vi "vipbBuild.vi"() -> (0 "error out":errorcluster)   [LabVIEW 2014, in "vipm-build-tools.lvlib"]
uses:
  vipm-build-tools.lvlib
  <vilib>/Utility/error.llb/DialogType.ctl
  <vilib>/Wiresmith Technology/LabVIEW CLI/CLI Class/CLI.lvclass
  <vilib>/JKI/VIPM API/VIPM API_vipm_api.lvlib
  build/lvcommonbuild.lvlib
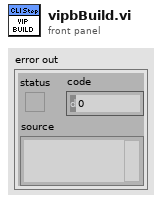
[diagram p1: front panel]
types:
  T1 = enum16{"open", "replace", "create", "open or create", "replace or create", "replace or create with confirmation"}
  T2 = typedef "DialogType.ctl" = u16
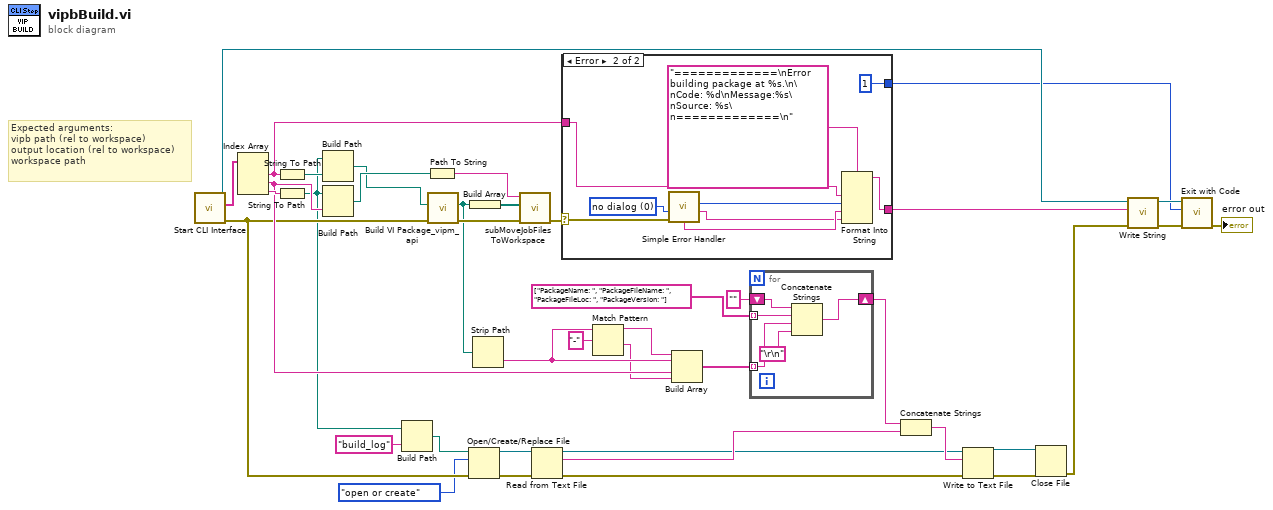
[diagram p0: block diagram]
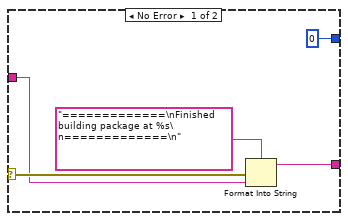
[diagram p2: hidden frame]
diagram:
  # "Expected arguments:\nvipb path (rel to workspace)\noutput location (rel to workspace)\nworkspace path"
  n1 = call <vilib>:"Start CLI Interface.vi"() -> ("error out"=w16:errorcluster, "Custom Parameters"=w40:string[], "CLI out"=w38:refnum<class "CLI.lvclass">)  [unwired: 9 in]
  n2 = Index Array(array=w40) -> (element #1=w20:string, element #2=w19:string, element #3=w32:string)  [unwired: 3 in]
  n3 = String To Path(string=w20) -> (path=w34:path)
  n4 = String To Path(string=w32) -> (path=w15:path)
  n5 = Build Path(base path=w15, name or relative path=w34) -> (appended path=w26:path)
  n6 = Build Path(base path=w15, name or relative path=w19) -> (appended path=w31:path)
  n7 = Build Path(base path=w15, name or relative path="build_log") -> (appended path=w13:path)
  n8 = Path To String(path=w31) -> (string=w28:string)
  n9 = call <vilib>:"Build VI Package_vipm_api.vi"("error in (no error)"=w16, "Path to VIPB File"=w26) -> ("error out"=w30:errorcluster, "Build Output"=w24:path)  [unwired: 8 in]
  n10 = Open/Create/Replace File(file path (use dialog)=w13, error in=w16, operation (0:open)=T1."open or create") -> (refnum out=w11:refnum<file>, error out=w10:errorcluster)  [unwired: 3 in, 1 out]
  n11 = Build Array(w24) -> (w27:path[])
  n12 = Strip Path(path=w24) -> (name=w21:string)  [unwired: 1 out]
  n13 = call "subMoveJobFilesToWorkspace.vi"("error in (no error)"=w30, "Generated Files"=w27, "Workspace Path"=w28) -> ("error out"=w29:errorcluster)  [unwired: 8 in]
  n14 = Read from Text File(file (use dialog)=w11, error in=w10) -> (refnum out=w5:refnum<file>, text=w7:string, error out=w4:errorcluster)  [unwired: 2 in, 1 out]
  n15 = case shown="Error" w29 {
    selector: w29 -> [w44 w53]
    tunnel: w20 -> [w43 w49]
    tunnel: [w42 w54] -> w39
    tunnel: [0 ("Exit Code (0)") 1 ("Exit Code (0)")] -> w35
    frame No Error {
      n16 = Format Into String(format string="=============\nFinished building package at %s\n=============\n", error in=w44, w43) -> (resulting string=w42:string)  [unwired: 1 in, 1 out]
    }
    frame Error {
      w52 = T2 0 items=["no dialog", "OK message", "continue or stop message", "OK message + warnings", "continue/stop + warnings"] ("type of dialog (OK msg:1)")
      n17 = call <vilib>:"Simple Error Handler.vi"("type of dialog (OK msg:1)"=w52, "error in (no error)"=w53) -> ("code out"=w46:i32, "source out"=w47:string, "message"=w48:string)  [unwired: 3 in, 2 out]
      n18 = Format Into String(format string="=============\nError building package at %s.\n\nCode: %d\nMessage:%s\nSource: %s\n=============\n", w49, w46, w48, w47) -> (resulting string=w54:string)  [unwired: 2 in, 1 out]
    }
  }
  n19 = Match Pattern(string=w21, regular expression="-") -> (before substring=w22:string, after substring=w18:string)  [unwired: 1 in, 2 out]
  n20 = Build Array(w22, w21, w19, w18) -> (w17:string[])
  n21 = for {
    tunnel: string[] ["PackageName: ", "PackageFileName: ", "PackageFileLoc: ", "PackageVersion: "] -> [w59] mode=indexing
    tunnel: w17 -> [w58] mode=indexing
    shift-right: [w56] -> w8
    shift-left: "" -> [w55]
    n22 = Concatenate Strings(w55, w59, w58, "\r\n") -> (w56:string)
  }
  n23 = Concatenate Strings(w8, w7) -> (w6:string)
  n24 = Write to Text File(file (use dialog)=w5, text=w6, error in=w4) -> (refnum out=w3:refnum<file>, error out=w2:errorcluster)  [unwired: 1 in, 1 out]
  n25 = Close File(refnum=w3, error in=w2) -> (error out=w1:errorcluster)  [unwired: 1 out]
  n26 = call <vilib>:"Write String.vi"("error in (no error)"=w1, "Text to Write"=w39, "CLI in"=w38) -> ("error out"=w37:errorcluster, "CLI out"=w36:refnum<class "CLI.lvclass">)  [unwired: 7 in]
  n27 = call <vilib>:"Exit with Code.vi"("error in (no error)"=w37, "Exit Code (0)"=w35, "CLI in"=w36) -> ("error out"=→"error out":errorcluster)  [unwired: 8 in]
